vi "Rename if exists.vi"(8 "error in":errorcluster, 11 "File Path":path) -> (0 "error out":errorcluster, 3 "New path":path)   [LabVIEW 2017]
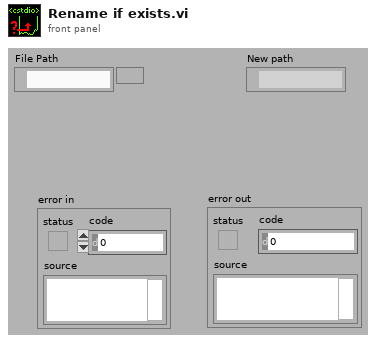
[diagram p1: front panel]
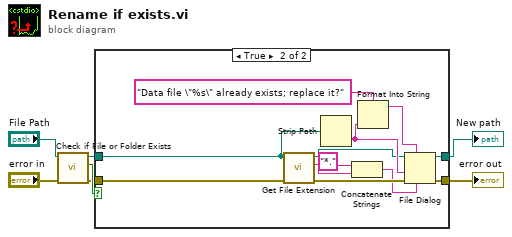
[diagram p0: block diagram]
diagram:
  n1 = call <vilib>:"Check if File or Folder Exists.vi"("error in (no error)"="error in", "path"="File Path") -> ("error out"=w4:errorcluster, "file or folder exists?"=w7:bool, "dup path"=w6:path)  [unwired: 7 out]
  n2 = case shown="True" w7 {
    tunnel: [w9 w17] -> w2
    tunnel: w4 -> [w9 w16]
    tunnel: [w8 w21] -> w3
    tunnel: w6 -> [w8 w14]
    frame False {
    }
    frame True {
      n3 = call <vilib>:"Get File Extension.vi"("error in (no error)"=w16, "file"=w14) -> ("error out"=w15:errorcluster, "lowercase file extension"=w12:string, "dup file"=w13:path)  [unwired: 7 out]
      n4 = Strip Path(path=w14) -> (name=w18:string)  [unwired: 1 out]
      n5 = Concatenate Strings("*." ("string"), w12) -> (w10:string)
      n6 = Format Into String(format string="Data file \"%s\" already exists; replace it?", w18) -> (resulting string=w19:string)  [unwired: 2 in, 1 out]
      n7 = File Dialog(6:w10, 7:w19, 8:w15, 9:w18, 11:w13) -> (0:w17:errorcluster, 3:w21:path)  [unwired: 4 out]
    }
  }
  "error out" <- w2
  "New path" <- w3
